vi "init.vi"(8 "error in (no error)":errorcluster, 11 "PicoMotor (in)":refnum<class "PicoMotor.lvclass">) -> (0 "error out":errorcluster, 2 "DeviceKey":string, 3 "PicoMotor":refnum<class "PicoMotor.lvclass">)   [LabVIEW 2013, in "PicoMotor.lvclass"]
uses:
  PicoMotor.lvclass
  PicoMotor.lvclass/PicoMotor.ctl
  Experiment/Globals.vi
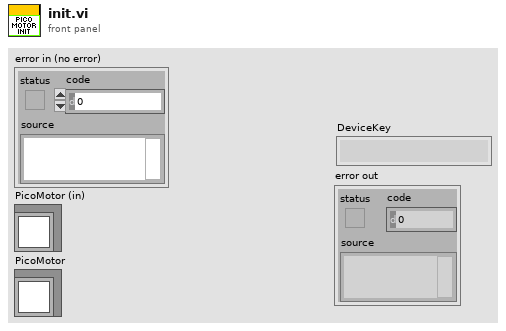
[diagram p1: front panel]
types:
  T1 = typedef "states.ctl" = enum16{"run", "pause", "shutdown gracefully", "halt immediately", "waiting for connection", "waiting for command"}
  T2 = typedef "PicoMotor.lvclass/picomotor_control_array.ctl" = T3[]
  T3 = typedef "PicoMotor.lvclass/picomotor_control.ctl" = cluster{"enable":bool, "description":string, "Set Position ":i32, "Actual Position":i32, "stopped?":bool, "zero":bool, "Motor Type":i32, "Steps/s":i32, "Steps/s^2":i32}
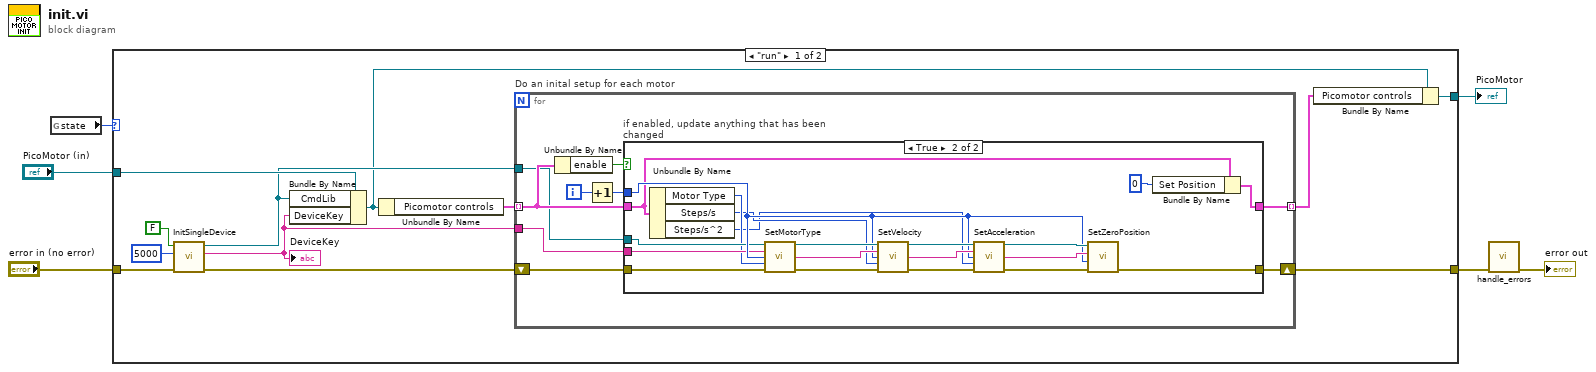
[diagram p0: block diagram]
diagram:
  n1 = global read "Globals.vi" "state"() -> (w3:T1)
  n2 = case shown="\"run\"" w3 {
    tunnel: [w8 w51] -> w5
    tunnel: "error in (no error)" -> [w16 w51]
    tunnel: "PicoMotor (in)" -> [w14 w50]
    tunnel: [w7 w50] -> w1
    frame "run" {
      n3 = call "InitSingleDevice.vi"("error in (no error)"=w16, "msecDelayForDiscovery"=5000, "logging"=FALSE) -> ("error out"=w11:errorcluster, "DeviceKey Out"=w12:string, "CmdLib Out"=w13:refnum<k24>)  [unwired: 2 in]
      "DeviceKey" <- w12
      n4 = Bundle By Name(cluster=w14, "CmdLib"=w13, "DeviceKey"=w12) -> (w10:refnum<class "PicoMotor.lvclass">)
      n5 = Unbundle By Name(w10) -> ("Picomotor controls"=w15:T2)
      n6 = for "Do an inital setup for each motor" {
        shift-right: [w25] -> w8
        shift-left: w11 -> [w24]
        tunnel: w15 -> [w23] mode=indexing
        tunnel: w13 -> [w22]
        tunnel: w12 -> [w21]
        tunnel: [w19] -> w9 mode=indexing
        i -> [w27]
        n7 = Unbundle By Name(w23) -> ("enable"=w20:bool)
        n8 = Increment(x=w27) -> (x+1=w26:i32)
        n9 = case "if enabled, update anything that has been changed" shown="True" w20 {
          tunnel: w24 -> [w29 w36]
          tunnel: w26 -> [_ w39]
          tunnel: [w29 w42] -> w25
          tunnel: w23 -> [w28 w32]
          tunnel: w22 -> [_ w38]
          tunnel: w21 -> [_ w37]
          tunnel: [w28 w30] -> w19
          frame False {
          }
          frame True {
            n10 = Unbundle By Name(w32) -> ("Motor Type"=w35:i32, "Steps/s"=w34:i32, "Steps/s^2"=w33:i32)
            n11 = call "SetMotorType.vi"("CmdLib In"=w38, "DeviceKey In"=w37, "Motor"=w39, "Motor Type"=w35, "error in (no error)"=w36) -> ("CmdLib Out"=w49:refnum<k24>, "DeviceKey Out"=w47:string, "error out"=w48:errorcluster)  [unwired: 8 in]
            n12 = call "SetVelocity.vi"("CmdLib In"=w49, "DeviceKey In"=w47, "Motor"=w39, "Steps Per Sec"=w34, "error in (no error)"=w48) -> ("CmdLib Out"=w44:refnum<k24>, "DeviceKey Out"=w45:string, "error out"=w46:errorcluster)  [unwired: 8 in]
            n13 = call "SetAcceleration.vi"("CmdLib In"=w44, "DeviceKey In"=w45, "Motor"=w39, "Steps Per Sec 2"=w33, "error in (no error)"=w46) -> ("CmdLib Out"=w41:refnum<k24>, "DeviceKey Out"=w40:string, "error out"=w43:errorcluster)  [unwired: 8 in]
            n14 = call "SetZeroPosition.vi"("error in (no error)"=w43, "Motor"=w39, "DeviceKey In"=w40, "CmdLib In"=w41) -> ("error out"=w42:errorcluster)  [unwired: 1 in, 2 out]
            n15 = Bundle By Name(cluster=w32, "Set Position"=0) -> (w30:T3)
          }
        }
      }
      n16 = Bundle By Name(cluster=w10, "Picomotor controls"=w9) -> (w7:refnum<class "PicoMotor.lvclass">)
    }
    frame Default {
    }
  }
  "PicoMotor" <- w1
  n17 = call "handle_errors.vi"("error in (no error)"=w5) -> ("error out"=→"error out":errorcluster)  [unwired: 14 in]
